vi "Actor Core.vi"(8 "error in":errorcluster, 11 "DT Controller in":refnum<class "DT Controller.lvclass">) -> (0 "error out":errorcluster, 3 "Actor out":refnum<class "Actor.lvclass">)   [LabVIEW 2019, in "DT Controller.lvlib" / "DT Controller.lvclass"]
doc: "(<B>Filename</B>: Actor Framework.lvlib:Actor.lvclass:Actor Core.vi)\n\nReceives messages to the actor, reacts to them, and initiates any error handling that may shut the actor down.\n\nDescendant classes may override this VI to append parallel tasks for the actor to complete while it handles messages. Overrides use the Call Parent Method node."
uses:
  DT Controller.lvclass
  C:/Program Files/National Instruments/LabVIEW 2019/vi.lib/ActorFramework/Actor/Actor.lvclass
  <vilib>/ActorFramework/Actor/Actor.lvclass
  DT GUI Plugin Manager/DT GUI Plugin Manager/DT GUI Plugin Manager.lvclass
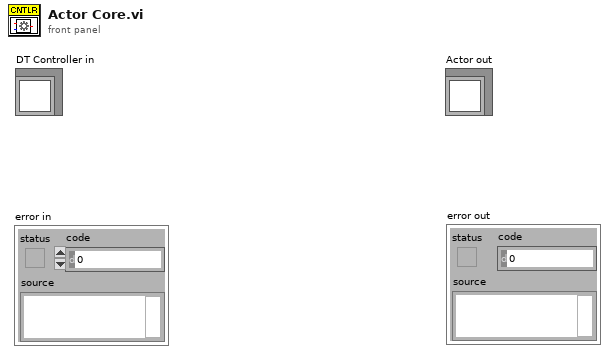
[diagram p1: front panel]
types:
  T1 = cluster{"DT GUI Plugin Manager.lvlib:DT GUI Plugin Manager.lvclass":refnum<class "DT GUI Plugin Manager.lvclass">, "Debug Alias":string}
  T2 = cluster{"DT GUI Plugin Manager.lvlib:DT GUI Plugin Manager.lvclass":refnum<class "DT GUI Plugin Manager.lvclass">, "Debug Alias":string}[]
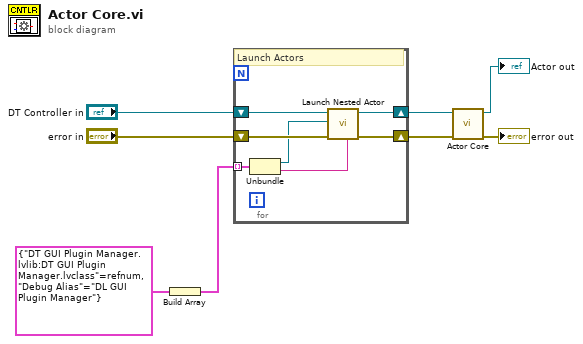
[diagram p0: block diagram]
diagram:
  n1 = Build Array(T1 {"DT GUI Plugin Manager.lvlib:DT GUI Plugin Manager.lvclass"=refnum, "Debug Alias"="DL GUI Plugin Manager"}) -> (w1:T2)
  n2 = for {
    shift-right: [w14] -> w5
    shift-left: "error in" -> [w15]
    shift-right: [w12] -> w3
    shift-left: "DT Controller in" -> [w13]
    tunnel: w1 -> [w11] mode=indexing
    # "Launch Actors"
    n3 = Unbundle(w11) -> ("DT GUI Plugin Manager.lvlib:DT GUI Plugin Manager.lvclass"=w10:refnum<class "DT GUI Plugin Manager.lvclass">, "Debug Alias"=w9:string)
    n4 = call <vilib>:"Launch Nested Actor.vi"("Debug Alias"=w9, "error in (no error)"=w15, "Nested Actor"=w10, "Caller Actor in"=w13) -> ("error out"=w14:errorcluster, "Caller Actor out"=w12:refnum<class "DT Controller.lvclass">)  [unwired: 5 in, 1 out]
  }
  n5 = call-parent "Actor Core.vi"("error in"=w5, "Actor in"=w3) -> ("error out"=→"error out":errorcluster, "Actor out"=→"Actor out":refnum<class "Actor.lvclass">)  [unwired: 8 in]
